vi "All analog data for display.vi"(11 "error inn":errorcluster) -> (8 "All analog data for graph":dbl[](array[numeric]), 15 "error out":errorcluster)   [LabVIEW 2011]
uses:
  Action Analog Handler.ctl
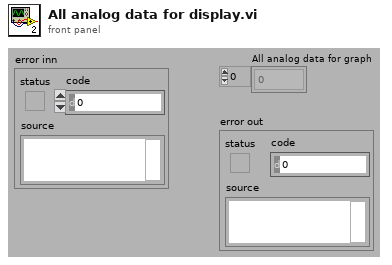
[diagram p1: front panel]
types:
  T1 = typedef "Action Analog Handler.ctl" = enum16{"GET value", "GET Single Frequenzy", "GET All Values", "GET Waveform", "Get Numb Var", "SET Value", "START Buffer", "REG Variable", "BUF size(total antal sekund)", "PULS", "Get a Value at time", "Set initial waveform"}
  T2 = typedef "User Setting Analog Channel Bg.ctl" = cluster{"Scaling":T3, "Limits and responces":T4, "Allow Graph selection by user":bool, "Unit":u16}
  T3 = typedef "Scaling.ctl" = cluster{"Gain":dbl, "Offset":dbl}
  T4 = typedef "Alarm Setup Analog.ctl" = cluster{"Technical Error(NA)":T5, "LL":T5, "L":T5, "H":T5, "HH":T5, "Limits":T7}
  T5 = typedef "Alarm Responce.ctl" = cluster{"Action":T6, "Alarm":bool}
  T6 = typedef "Action List.ctl" = enum16{"No Action", "Stop Motor", "Turn Off HV"}
  T7 = typedef "Limits.ctl" = cluster{"LL":dbl, "L":dbl, "H":dbl, "HH":dbl}
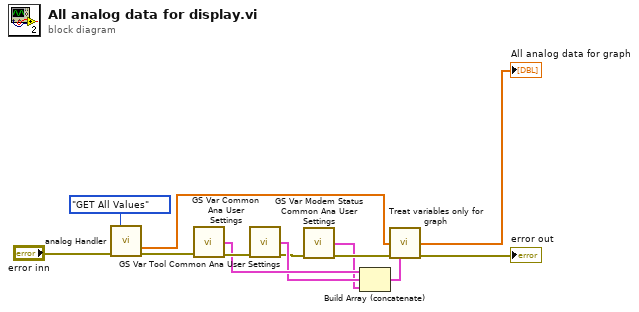
[diagram p0: block diagram]
diagram:
  n1 = call "analog Handler.vi"("Action"=Action_Analog_Handler."GET All Values" ("Action(GET)"), "error in (no error)"="error inn") -> ("Values"=w6:dbl[], "error out"=w11:errorcluster)  [unwired: 8 in, 4 out]
  n2 = call "GS Var Common Ana User Settings.vi"("error in (no error)"=w11) -> ("Common Analog var User set out"=w9:T2[], "error out"=w10:errorcluster)  [unwired: 12 in, 1 out]
  n3 = call "GS Var Tool Common Ana User Settings.vi"("error in (no error)"=w10) -> ("Tool Analog var User settigns out"=w8:T2[], "error out"=w3:errorcluster)  [unwired: 12 in, 1 out]
  n4 = call "GS Var Modem Status Common Ana User Settings.vi"("error in (no error)"=w3) -> ("Modem Status Analog var User settigns out"=w1:T2[], "error out"=w2:errorcluster)  [unwired: 12 in, 1 out]
  n5 = Build Array (concatenate)(w9, w8, w1) -> (w7:T2[])
  n6 = call "Treat variables only for graph.vi"("Analog values"=w6, "error In"=w2, "Analog Variable info Settings"=w7) -> ("Analog Values"=→"All analog data for graph":dbl[], "error out"=→"error out":errorcluster)  [unwired: 11 in]
